vi "Start Dispatcher.vi"(0 "UDP port (0)":u16, 5 "use any port (F)":bool, 11 "error in":errorcluster) -> (4 "UDP port used":u16, 6 "execution state before start":T1(ring), 15 "error out":errorcluster)   [LabVIEW 2015, in "TLB` Template.lvlib" / "AMC.lvlib"]
doc: "Asynchronously launches the Dispatcher process, which receives AMC messages sent from other application instances.\n\nIf \"UDP port\" is undefined and \"use any port\" is True, the Dispatcher will use any available port.\nIf \"UDP port\" is undefined and \"use any port\" is False, the Dispatcher will use the default port.\nIf \"UDP port\" is defined, the Dispatcher will use that port.TLB Prime - Application Template 1.3.0.24\nNorm Kirchner, NI Systems Engineering - NI\nCopyright (c) 2014, NI"
uses:
  AMC.lvlib
  FG Dispatcher Status.vi
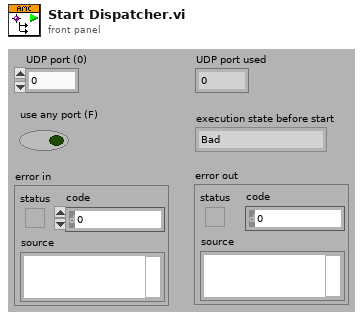
[diagram p1: front panel]
types:
  T1 = enum32{"Bad", "Idle", "Run top level", "Running"}
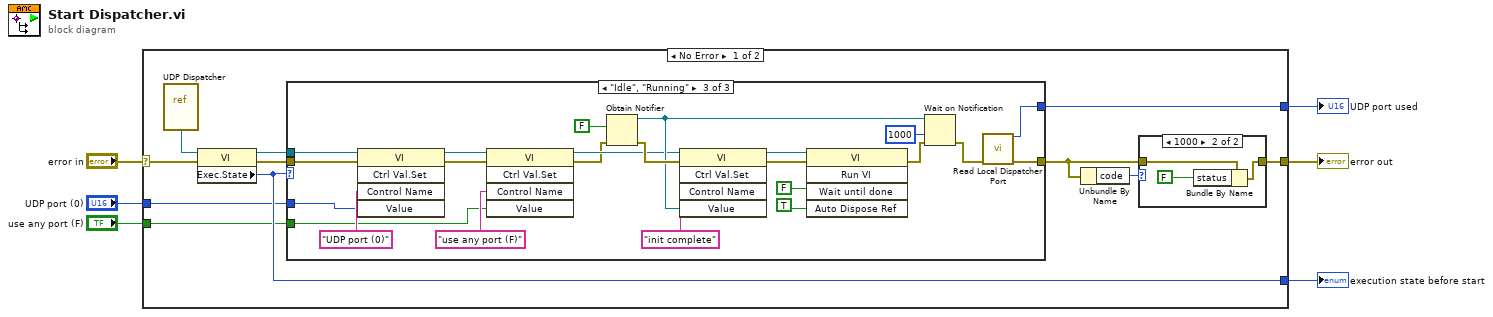
[diagram p0: block diagram]
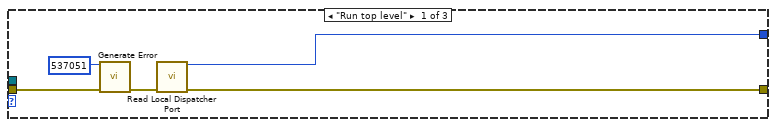
[diagram p2: hidden frame]
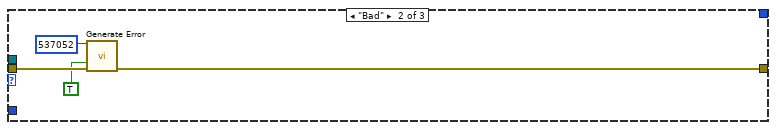
[diagram p3: hidden frame]
diagram:
  n1 = case shown="No Error" "error in" {
    selector: "error in" -> [w11 w54]
    tunnel: [w16 w54] -> w6
    tunnel: [w12 _] -> w4
    tunnel: "UDP port (0)" -> [w9 _]
    tunnel: [w8 _] -> w2
    tunnel: "use any port (F)" -> [w7 _]
    frame No Error {
      n2 = vi-ref "UDP Dispatcher.vi"() -> (w10:refnum<vi>)
      n3 = property class="VI"(reference=w10, error in=w11) -> (reference out=w15:refnum<vi>, error out=w14:errorcluster, "Exec.State"=w12:T1)
      n4 = case shown="\"Idle\", \"Running\"" w12 {
        tunnel: [w19 w24 w34] -> w13
        tunnel: w15 -> [_ _ w47]
        tunnel: w14 -> [w21 w25 w46]
        tunnel: w9 -> [_ _ w44]
        tunnel: [w18 _ w33] -> w8
        tunnel: w7 -> [_ _ w27]
        frame "Run top level" {
          n5 = call "Generate Error.vi"("code"=537051, "error in"=w21) -> ("error out"=w20:errorcluster)  [unwired: 13 in]
          n6 = call "Read Local Dispatcher Port.vi"("error in"=w20) -> ("UDP port"=w18:u16, "error out"=w19:errorcluster)  [unwired: 13 in]
        }
        frame "Bad" {
          n7 = call "Generate Error.vi"("code"=537052, "status (F)"=TRUE, "error in"=w25) -> ("error out"=w24:errorcluster)  [unwired: 12 in]
        }
        frame "Idle", "Running" {
          n8 = invoke class="VI" method="Ctrl Val.Set"(reference=w47, error in=w46, "Control Name"="UDP port (0)", "Value"=w44) -> (reference out=w32:refnum<vi>, error out=w30:errorcluster)  [unwired: 1 in, 3 out]
          n9 = invoke class="VI" method="Ctrl Val.Set"(reference=w32, error in=w30, "Control Name"="use any port (F)", "Value"=w27) -> (reference out=w31:refnum<vi>, error out=w29:errorcluster)  [unwired: 1 in, 3 out]
          n10 = Obtain Notifier(notification data type=FALSE, error in (no error)=w29) -> (notifier out=w38:refnum<notifier>, error out=w39:errorcluster)  [unwired: 2 in, 1 out]
          n11 = invoke class="VI" method="Ctrl Val.Set"(reference=w31, error in=w39, "Control Name"="init complete", "Value"=w38) -> (reference out=w43:refnum<vi>, error out=w42:errorcluster)  [unwired: 1 in, 3 out]
          n12 = invoke class="VI" method="Run VI"(reference=w43, error in=w42, "Wait until done"=FALSE ("Wait Until Done"), "Auto Dispose Ref"=TRUE) -> (error out=w37:errorcluster)  [unwired: 1 in, 4 out]
          n13 = Wait on Notification(notifier=w38, timeout in ms (-1)=1000, error in (no error)=w37) -> (error out=w35:errorcluster)  [unwired: 1 in, 3 out]
          n14 = call "Read Local Dispatcher Port.vi"("error in"=w35) -> ("UDP port"=w33:u16, "error out"=w34:errorcluster)  [unwired: 13 in]
        }
      }
      n15 = Unbundle By Name(w13) -> ("code"=w17:i32)
      n16 = case shown="1000" w17 {
        tunnel: w13 -> [w50 w53]
        tunnel: [w50 w52] -> w16
        frame 0, Default {
        }
        frame 1000 {
          n17 = Bundle By Name(cluster=w53, "status"=FALSE) -> (w52:errorcluster)
        }
      }
    }
    frame Error {
    }
  }
  "error out" <- w6
  "execution state before start" <- w4
  "UDP port used" <- w2
